vi "test_Multiple Global and Local MetaData Single and Array Channel Command-Response Messages using Trigger and Padding.vi"(8 "error in (no error)":errorcluster, 11 "TestCase in":refnum<class "Instrument Addon Common System Tests.lvclass">) -> (0 "error out":errorcluster, 3 "TestCase out":refnum<class "Instrument Addon Common System Tests.lvclass">)   [LabVIEW 2018, in "Instrument Addon Common System Tests.lvclass"]
uses:
  Instrument Addon Common System Tests.lvclass
  C:/Dev/niveristand-custom-device-testing-tools/VeriStandTestCase/VeriStandTestCase.lvclass
  <vilib>/NI Veristand/Execution/Workspace/NI VeriStand - Set Multiple Channel Values.vi
  <vilib>/NI Veristand/Execution/Workspace/NI VeriStand - Get Multiple Channel Values.vi
  <vilib>/addons/_JKI Toolkits/VI Tester/TestCase.llb/TestCase.lvclass
  <vilib>/NI Veristand/Execution/Workspace/NI_VS Workspace ExecutionAPI.lvlib
  C:/Program Files (x86)/National Instruments/LabVIEW 2018/vi.lib/addons/_JKI Toolkits/VI Tester/TestCase.llb/TestCase.lvclass
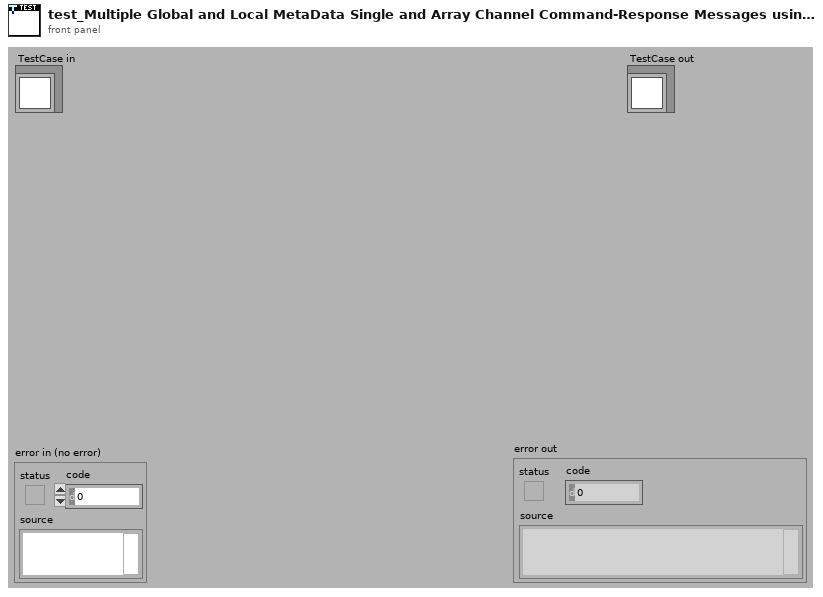
[diagram p1: front panel]
types:
  T1 = typedef "NI_VS Workspace ExecutionAPI.lvlib/WorkspaceAPI.ctl" = refnum<k24>
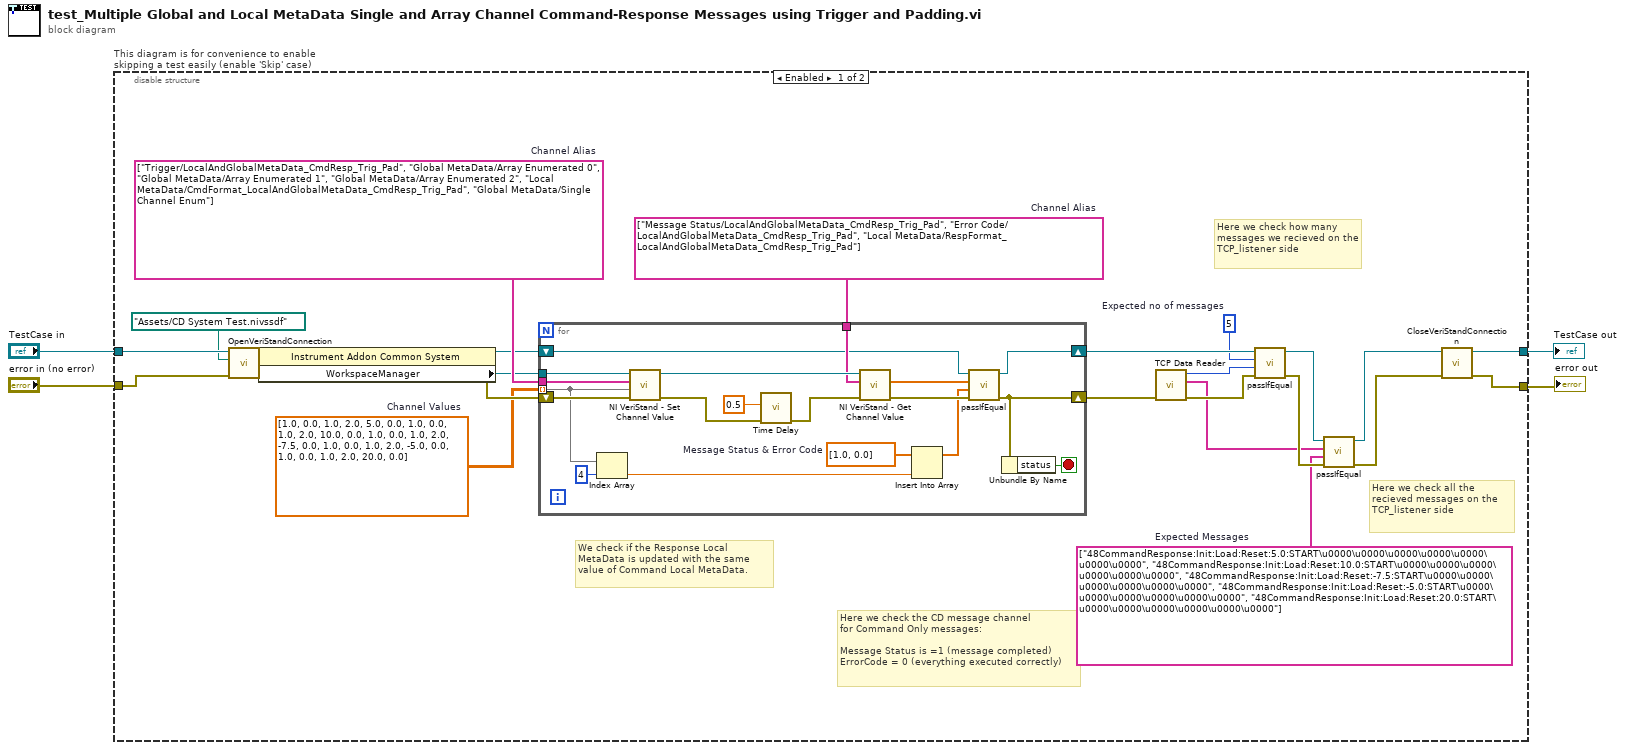
[diagram p0: block diagram]
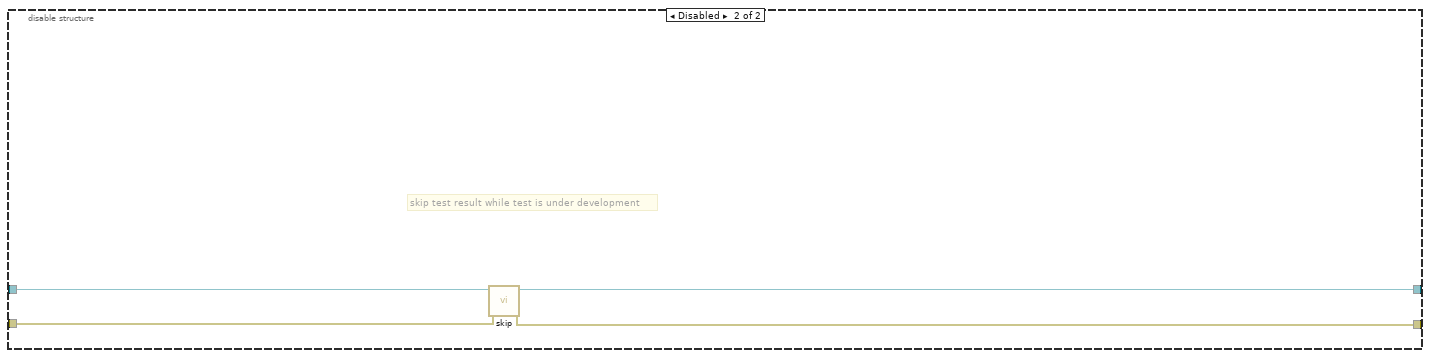
[diagram p2: hidden frame]
diagram:
  n1 = disable-structure "This diagram is for convenience to enable skipping a test easily (enable 'Skip' case)" shown="Enabled" {
    disable-tunnel: "TestCase in" -> [w26 w51]
    disable-tunnel: [w27 w49] -> w1
    disable-tunnel: [w28 w50] -> w3
    disable-tunnel: "error in (no error)" -> [w24 w48]
    frame Enabled {
      w5 = string[] ["48CommandResponse:Init:Load:Reset:5.0:START\u0000\u0000\u0000\u0000\u0000\u0000\u0000", "48CommandResponse:Init:Load:Reset:10.0:START\u0000\u0000\u0000\u0000\u0000\u0000", "48CommandResponse:Init:Load:Reset:-7.5:START\u0000\u0000\u0000\u0000\u0000\u0000", "48CommandResponse:Init:Load:Reset:-5.0:START\u0000\u0000\u0000\u0000\u0000\u0000", "48CommandResponse:Init:Load:Reset:20.0:START\u0000\u0000\u0000\u0000\u0000\u0000"]  # Expected Messages
      w8 = 5  # Expected no of messages
      w17 = string[] ["Message Status/LocalAndGlobalMetaData_CmdResp_Trig_Pad", "Error Code/LocalAndGlobalMetaData_CmdResp_Trig_Pad", "Local MetaData/RespFormat_LocalAndGlobalMetaData_CmdResp_Trig_Pad"]  # Channel Alias
      w19 = dbl[][] [[1.0, 0.0, 1.0, 2.0, 5.0, 0.0], [1.0, 0.0, 1.0, 2.0, 10.0, 0.0], [1.0, 0.0, 1.0, 2.0, -7.5, 0.0], [1.0, 0.0, 1.0, 2.0, -5.0, 0.0], [1.0, 0.0, 1.0, 2.0, 20.0, 0.0]]  # Channel Values
      w20 = string[] ["Trigger/LocalAndGlobalMetaData_CmdResp_Trig_Pad", "Global MetaData/Array Enumerated 0", "Global MetaData/Array Enumerated 1", "Global MetaData/Array Enumerated 2", "Local MetaData/CmdFormat_LocalAndGlobalMetaData_CmdResp_Trig_Pad", "Global MetaData/Single Channel Enum"]  # Channel Alias
      # "We check if the Response Local MetaData is updated with the same value of Command Local MetaData."
      # "Here we check how many messages we recieved on the TCP_listener side"
      # "Here we check all the recieved messages on the TCP_listener side"
      # "Here we check the CD message channel\nfor Command Only messages:\n\nMessage Status is =1 (message completed)\nErrorCode = 0 (everything executed correctly)"
      n2 = call-dynamic "OpenVeriStandConnection.vi"("error in (no error)"=w24, "System Definition File"=path "Assets/CD System Test.nivssdf", "VeriStand Test Case in"=w26) -> ("error out"=w23:errorcluster, "VeriStand Test Case out"=w25:refnum<class "Instrument Addon Common System Tests.lvclass">)  [unwired: 6 in, 1 out]
      n3 = property class="Instrument Addon Common System "(reference=w25, error in=w23) -> (reference out=w18:refnum<class "Instrument Addon Common System Tests.lvclass">, error out=w21:errorcluster, "WorkspaceManager"=w16:T1)
      n4 = for {
        tunnel: w16 -> [w47]
        tunnel: w20 -> [w45]
        tunnel: w19 -> [w31] mode=indexing
        shift-right: [w34] -> w7
        shift-left: w21 -> [w46]
        tunnel: w17 -> [w43]
        shift-right: [w38] -> w15
        shift-left: w18 -> [w39]
        stop <- w33 stop-if-true
        w35 = dbl[] [1.0, 0.0]  # Message Status & Error Code
        n5 = Index Array(array=w31, index=4) -> (element=w29:dbl)
        n6 = call-poly <vilib>:"NI VeriStand - Set Channel Value.vi"("error in (no error)"=w46, "Values"=w31, "Channels"=w45, "WorkspaceManager in"=w47) -> ("error out"=w41:errorcluster, "WorkspaceManager out"=w44:T1)  [unwired: 6 in]
        n7 = call "Time Delay"("error in (no error)"=w41, "Delay Time (s)"=0.5) -> ("error out"=w40:errorcluster)  [unwired: 9 in]
        n8 = call-poly <vilib>:"NI VeriStand - Get Channel Value.vi"("error in (no error)"=w40, "Channels"=w43, "WorkspaceManager in"=w44) -> ("error out"=w37:errorcluster, "Values"=w36:dbl[])  [unwired: 6 in, 1 out]
        n9 = Insert Into Array(array=w35, new element=w29) -> (w32:dbl[])  [unwired: 1 in]
        n10 = call-dynamic "passIfEqual.vi"("error in (no error)"=w37, "y"=w32, "x"=w36, "TestCase in"=w39) -> ("error out"=w34:errorcluster, "TestCase out"=w38:refnum<class "Instrument Addon Common System Tests.lvclass">)  [unwired: 6 in]
        n11 = Unbundle By Name(w34) -> ("status"=w33:bool)
      }
      n12 = call "TCP Data Reader.vi"("error in (no error)"=w7) -> ("error out"=w13:errorcluster, "Recieved Messages"=w6:string[], "No of messages"=w9:i32)  [unwired: 8 in]
      n13 = call-dynamic "passIfEqual.vi"("error in (no error)"=w13, "y"=w9, "x"=w8, "TestCase in"=w15) -> ("error out"=w11:errorcluster, "TestCase out"=w14:refnum<class "Instrument Addon Common System Tests.lvclass">)  [unwired: 6 in]
      n14 = call-dynamic "passIfEqual.vi"("error in (no error)"=w11, "y"=w5, "x"=w6, "TestCase in"=w14) -> ("error out"=w10:errorcluster, "TestCase out"=w12:refnum<class "Instrument Addon Common System Tests.lvclass">)  [unwired: 6 in]
      n15 = call-dynamic "CloseVeriStandConnection.vi"("error in (no error)"=w10, "VeriStand Test Case in"=w12) -> ("error out"=w28:errorcluster, "VeriStand Test Case out"=w27:refnum<class "Instrument Addon Common System Tests.lvclass">)  [unwired: 8 in]
    }
    frame Disabled {
      # "skip test result while test is under development"
      n16 = call <vilib>:"skip.vi"("error in (no error)"=w48, "TestCase in"=w51) -> ("error out"=w50:errorcluster, "TestCase out"=w49:refnum<class "Instrument Addon Common System Tests.lvclass">)  [unwired: 8 in]
    }
  }
  "error out" <- w3
  "TestCase out" <- w1
